vi "Reas HAL Config Data.vi"(8 "error in (no error)":errorcluster, 11 "MSX-E3711 in":refnum<class "MSX-E3711.lvclass">) -> (0 "error out":errorcluster, 3 "MSX-E3711 out":refnum<class "MSX-E3711.lvclass">)   [LabVIEW 2014, in "MSX-E3711.lvclass"]
uses:
  MSX-E3711.lvclass
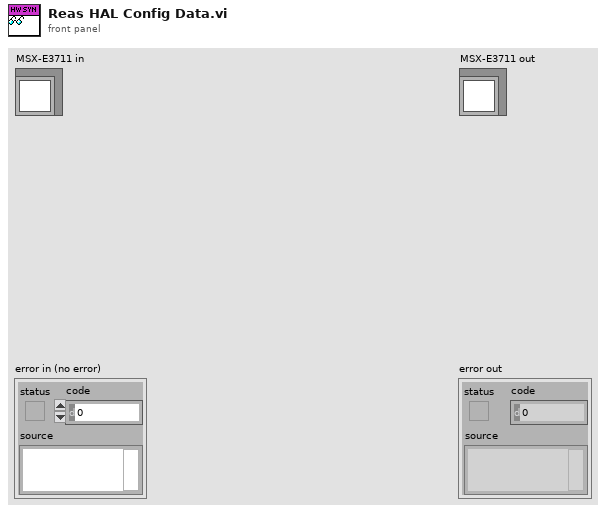
[diagram p1: front panel]
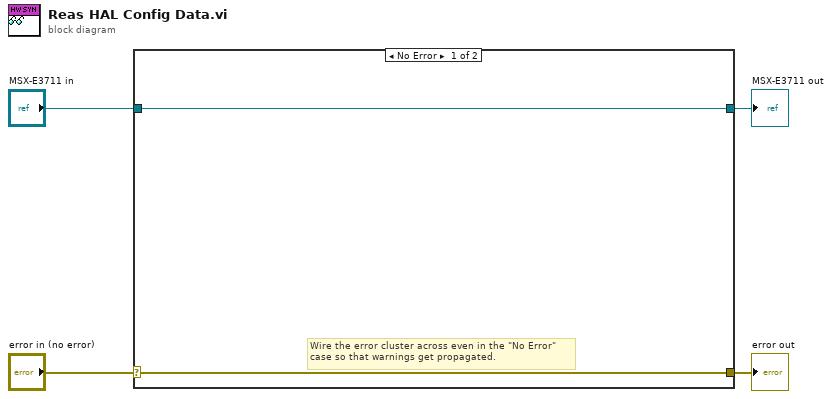
[diagram p0: block diagram]
diagram:
  n1 = case shown="No Error" "error in (no error)" {
    selector: "error in (no error)" -> [w5 w8]
    tunnel: [w5 w8] -> w3
    tunnel: [w6 w7] -> w1
    tunnel: "MSX-E3711 in" -> [w6 w7]
    frame No Error {
      # "Wire the error cluster across even in the \"No Error\"\ncase so that warnings get propagated."
    }
    frame Error {
    }
  }
  "error out" <- w3
  "MSX-E3711 out" <- w1
